vi "derive weighted array.vi"(10 "Full transition sequence from service to end":string[](array[string])=["-2 0 3 0 -3 0 4 -4 0\r\n", "0 3\r\n", "0 4 -3 0 -4 1 0 4 -3 0\r\n", "0\r\n", "-2 0 3 -3 0 -4 1 -4 0 3 -3 4 -3 0 2 0 3\r\n", "0 3 0 1\r\n", "0 1 0 3\r\n", "0 3 -2 0 4\r\n", "0\r\n", "0 -3 4 0 2 -2 0 -3 0 3 -2 3 -3 4\r\n", "0 -3 4 -3 0\r\n", "-2 0 -2 2 0\r\n", "0 3 -2\r\n", "0 4 -3 0 3 -2 0 -3 4 -3 0 3 -2 2 -2 0 4 0\r\n", "2 0 1 -4 0 3 0 -4 4 0 -4 4 0 2 0 4 0 -3 4 -3 0 -4 0 4\r\n", "0 4\r\n", "-2 0 -2 0 3 0\r\n", "0 3 0 -2 3\r\n", "0 4 0 4 -4 0 2 0 -4 4 -3 0 -2 2 -2 0 4 -3 0 2 0 3 0\r\n", "0 4 -3 0 1 -1 0 3 0 -2 2 -2 0 -3 4 -3 0 4 -4 1 0\r\n", "", "0 -3\r\n", "2 0 3 0 1 0 -2 3\r\n", "0\r\n", "1 -1 0\r\n", "0 -2 3 0\r\n", "0 1 0 4 0 4 -4 4\r\n", "0 1 -1 0 3\r\n", "0 2 -2 3 -3 4\r\n", "-2 2 0 -2 3\r\n", "0 -1\r\n", "0 4 -4 4 0 3 0 -2 0 -4 0 1 -4\r\n", "-2 0 4 0 -3 3 0 -2 2 -2 0 -4 0 4 0\r\n", "0 -1 0 -4 4 -4 1 -4 0\r\n", "1 -4 1 0 2 0 -3 0 2 0 -2 0 1 0 1 -4 4 -4 1 0 3 -2 0 -4 4 -4\r\n", "0 1 -4 4 -4 1\r\n", "0 3 0 -3 3 0 1 0 1 -4 4\r\n", "0 1 -4 0 1 -4\r\n", "0 3 -2 0 1 -4 1 0 2 0 4 0 4 0 -1 2 -1 0\r\n", "1 0 -1 0 2 0 4 -4\r\n", "-4\r\n", "-1 0 4\r\n", "0 1 -1 0 1 -4 0\r\n", "-1 0 1 -4 0 3 0 2 0 4 0 -4 4 -4 0 -1 0 -4 0 -2 0 4\r\n", "0 4 0\r\n", "0 4 -4 0 2 -1 0 2 0 4 -4 1 -4 4 0 3\r\n", "0 4 0 2 0\r\n", "1 0 -1 1 0 -4 1 -4 1 0 -4\r\n", "0 3 -2 0 -4\r\n", "2 -1 0 -4 4 -4 0 2 0 4\r\n", "1 0\r\n", "-1 0 -1 1 0 -4\r\n", "0 3 0\r\n", "0 -4 4 -4 0 -4 0 4 0 2 0 1 -4 4\r\n", "-1 0 1 -4\r\n", "-1 0 2 -1 0 2\r\n", "1 -1 0 4 -4 1\r\n", "-1 0 1 -4 4 -4 0 -4 4\r\n", "0 3 0 3 0 1 -1 0 1\r\n", "-1 0 4 0 4 -4 1 0 -4 0\r\n", "1 0 4\r\n", "0 -1 0 2 -1 0 -2 3 -2 0 -4 4 -4\r\n", "0 3 0\r\n", "2 -1 0 1 -4 4 -4 0 2 0\r\n", "0 4 -4 1 0 1 0 1 -4 0 2 0 4 0 4 -4 1\r\n", "1 -1 0 3 0 3 0 1 0 4\r\n", "0 -4 0 -2 0 -4\r\n", "0 -4 4 -4 0 -2 0 2 0\r\n", "-1 0 4 -4 0\r\n", "1 0 -1 2 0 4\r\n", "0 2 0 -2 0\r\n", "0 1 -4 0 -4 0 3 -2 0 -4 0 -4 4 -4 1\r\n", "0 4 0 4 0 4 0 4 0 -2 3 0 3 0 4 0\r\n", "-4 -1\r\n", "-2 0 1 0 -4 4\r\n", "0 4\r\n", "-2 2 0 -1 -4 1 0 3 0\r\n", "-1 0 -1 2\r\n", "0 -1 1 0 4 0 3 -2 0 -2 3 -2 0 4 0 -2 2\r\n", "2 -1 0 4\r\n", "0 4 0 2 0 -2 0\r\n", "1 -1 0 3 0 -4 4 -4 0\r\n", "2 -1 0 3 -2 0 -3 0 3 0 -3 0\r\n", "0 4 0 4 -4 1 -1 0 -3 0 1 -4 1 0 4 0 -4 0 -4 4 -4 1\r\n", "0 -4 1 0 -4 4\r\n", "0 4 0 -2 2 -2 2 -2 2\r\n", "-2 2 -1 0 4 0 2 0 4 0 2 -2 0 4\r\n", "1 0 -1 0 -1 0 1 -1\r\n", "-2 2 -2 3\r\n", "1 0 -1 0 -1 2 0 2 -2 0 -4 0\r\n", "-2 2 0 3 -2 2\r\n", "0\r\n", "1 -1 0 3\r\n", "0 4 0\r\n", "-2 0 1 -4 0 -3 0\r\n", "1 0 -1 2 -1 1 -4\r\n", "0 4\r\n", "-2 0 -1 1\r\n", "0 3 0 3 0 3 -2\r\n", "-4 0 -4 4\r\n", "0 4 0 -4 0 -4\r\n", "-2 2 0 4 -4 0 2 -2\r\n", "-2 2 -2 0 -1\r\n", "0 4 -3 0\r\n", "0 1 0 -1 1\r\n", "-4 0\r\n", "-2 0 3 0 1 0 3 -2 0 -1 0 4 0 3 0 -3 3 -3\r\n", "0 4 0 -2 0 1 0 -4 4 -3 0 1 0 4 0 -4 1 0 3 -3 0\r\n", "0 -1 2\r\n", "2 0 -3 4 0\r\n", "-4 0 -3 3 -3 0 -3 3 0 -2 3 0\r\n", "0 -1 1 -4 4 -3 0 3 0\r\n", "0 -1 2 0 3 0 1 -4 4 0 2 0\r\n", "2 -2 0 -4 0 -4 4 0 -4\r\n", "1 -1 2 -1\r\n", "2 0 -2 0 4 0 2 0 3 0 -2 0 -4\r\n", "1 -1 0 -1\r\n", "0 1 -4 1\r\n", "0 4 0 -1 1 -1 0\r\n", "0 3\r\n", "-2 0\r\n", "1 -4 0 -2 0 4 0 -4 0 4 -3 0 1 -4 0 1\r\n", "0 -3 3 -2 0 3 0 -2 2\r\n", "1 0\r\n", "2\r\n", "0 -4\r\n", "0 4 0 -4 0 -3 3 -3 0 -2 0 -2 0 4 0 -1 1 0 3 0 -4 1 -4 0 4\r\n", "2 0 -1 1\r\n", "0 2 0 4 0 4 -4 0 -1 2\r\n", "0 3 -2 0 3 -2\r\n", "1 0 -3 3 0 -4\r\n", "0 -3 3 0 -1 0\r\n", "2 -2 0 1\r\n", "-4 1 -4 1 -4 0\r\n", "0 4 0 2 0 -4 1 2 -1 0 4 0 1 0 4 -4 4 0 -4 4 0\r\n", "-2 0 3 0 -2 0\r\n"]) -> (2 "Weighted arrays":dbl[][][](array[numeric]))   [LabVIEW 2014]
panel:
  out "averaged weights":dbl[][](array[numeric])
  out "total weights":i32[][](array[numeric])
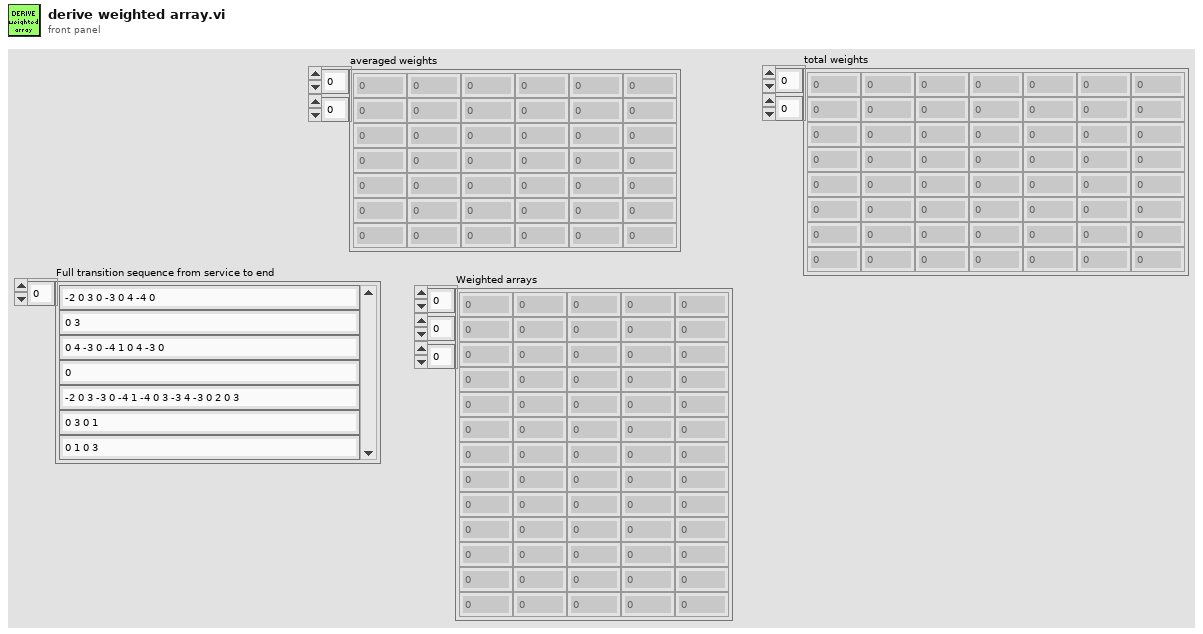
[diagram p1: front panel]
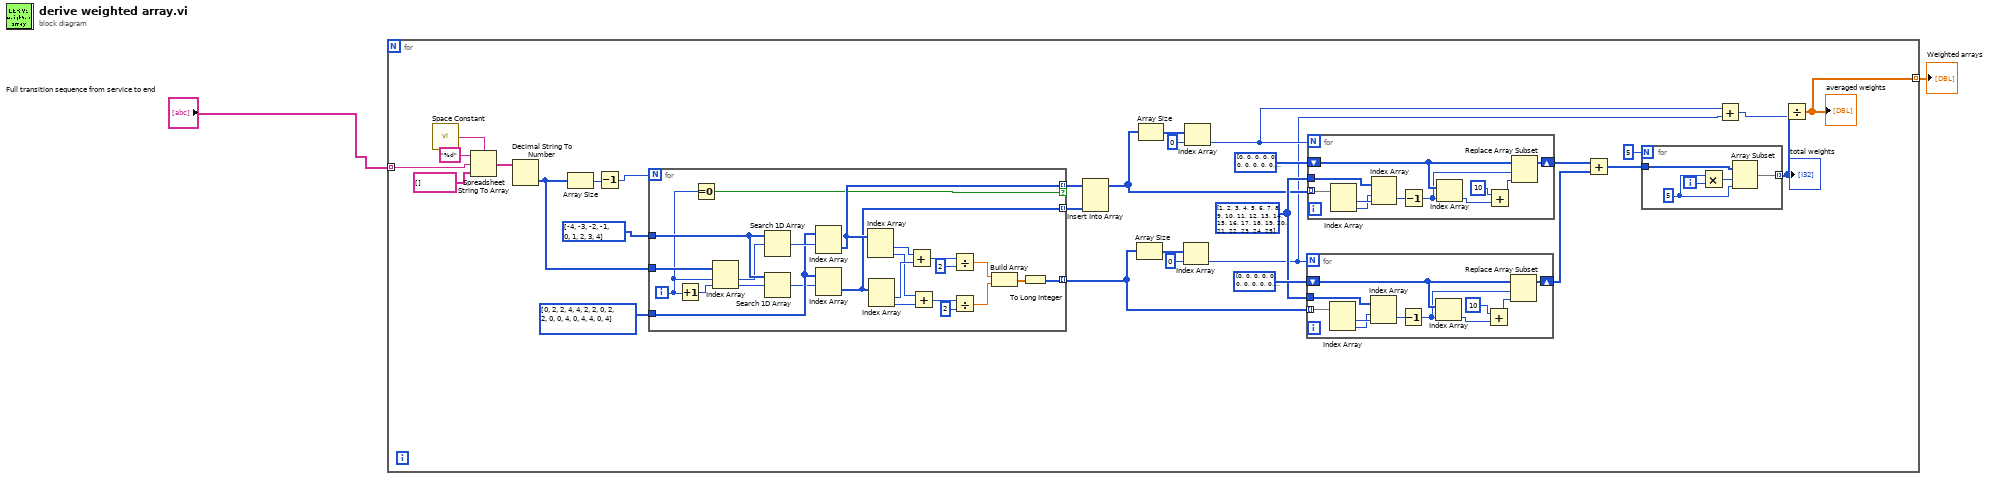
[diagram p0: block diagram]
diagram:
  n1 = for {
    tunnel: "Full transition sequence from service to end" -> [w4] mode=indexing
    tunnel: [w3] -> w1 mode=indexing
    w16 = i32[][] [[1, 2, 3, 4, 5], [6, 7, 8, 9, 10], [11, 12, 13, 14, 15], [16, 17, 18, 19, 20], [21, 22, 23, 24, 25]]
    n2 = call <vilib>:"Space Constant.vi"() -> ("String"=w32:string)
    n3 = Spreadsheet String To Array(delimiter (Tab)=w32, format string="%d", spreadsheet string=w4, array type (2D Dbl)=string[] []) -> (array=w29:string[])
    n4 = Decimal String To Number(string=w29) -> (number=w26:i32[])  [unwired: 2 in, 1 out]
    n5 = Array Size(array=w26) -> (size(s)=w28:i32)
    n6 = Decrement(x=w28) -> (x-1=w27:i32)
    n7 = for {
      N: w27 -> [_]
      tunnel: w26 -> [w82]
      tunnel: i32[] [-4, -3, -2, -1, 0, 1, 2, 3, 4] ("deleted portion") -> [w81]
      tunnel: i32[][] [[0, 2], [2, 4], [4, 2], [2, 0], [2, 2], [0, 0], [4, 0], [4, 4], [0, 4]] -> [w77]
      tunnel: [w62] -> w15 mode=indexing
      tunnel: [w63] -> w12 mode=indexing
      tunnel: [w65] -> w13 mode=indexing if=w61
      i -> [w60]
      n8 = Increment(x=w60) -> (x+1=w83:i32)
      n9 = Equal To 0?(x=w60) -> (x = 0?=w61:bool)
      n10 = Index Array(array=w82, index #1=w60, index #2=w83) -> (element #1=w80:i32, element #2=w79:i32)
      n11 = Search 1D Array(1D array=w81, element=w80) -> (index of element=w78:i32)  [unwired: 1 in]
      n12 = Search 1D Array(1D array=w81, element=w79) -> (index of element=w76:i32)  [unwired: 1 in]
      n13 = Index Array(array=w77, index (row)=w78) -> (element=w65:i32[])  [unwired: 1 in]
      n14 = Index Array(array=w77, index (row)=w76) -> (element=w63:i32[])  [unwired: 1 in]
      n15 = Index Array(array=w65) -> (element #1=w75:i32, element #2=w73:i32)  [unwired: 2 in]
      n16 = Index Array(array=w63) -> (element #1=w74:i32, element #2=w72:i32)  [unwired: 2 in]
      n17 = Add(x=w75, y=w74) -> (x+y=w71:i32)
      n18 = Add(x=w73, y=w72) -> (x+y=w68:i32)
      n19 = Divide(x=w71, y=2) -> (x/y=w67:dbl)
      n20 = Divide(x=w68, y=2) -> (x/y=w66:dbl)
      n21 = Build Array(w67, w66) -> (w64:dbl[])
      n22 = To Long Integer(number=w64) -> (32bit integer=w62:i32[])
    }
    n23 = Insert Into Array(array=w13, new element=w12) -> (w14:i32[][])  [unwired: 2 in]
    n24 = Array Size(array=w15) -> (size(s)=w18:i32[])
    n25 = Array Size(array=w14) -> (size(s)=w22:i32[])
    n26 = Index Array(array=w18, index=0) -> (element=w5:i32)
    n27 = Index Array(array=w22, index=0) -> (element=w6:i32)
    n28 = for {
      N: w5 -> [_]
      tunnel: w15 -> [w43] mode=indexing
      tunnel: w16 -> [w42]
      shift-right: [w34] -> w11
      shift-left: i32[] [0, 0, 0, 0, 0, 0, 0, 0, 0, 0, 0, 0, 0, 0, 0, 0, 0, 0, 0, 0, 0, 0, 0, 0, 0] -> [w36]
      n29 = Index Array(array=w43) -> (element #1=w41:i32, element #2=w40:i32)  [unwired: 2 in]
      n30 = Index Array(array=w42, index (row)=w40, index (col)=w41) -> (element=w39:i32)
      n31 = Decrement(x=w39) -> (x-1=w35:i32)
      n32 = Index Array(array=w36, index=w35) -> (element=w38:i32)
      n33 = Add(x=10, y=w38) -> (x+y=w37:i32)
      n34 = Replace Array Subset(array=w36, new element=w37, index=w35) -> (w34:i32[])
    }
    n35 = for {
      N: w6 -> [_]
      tunnel: w14 -> [w59] mode=indexing
      tunnel: w16 -> [w58]
      shift-right: [w50] -> w10
      shift-left: i32[] [0, 0, 0, 0, 0, 0, 0, 0, 0, 0, 0, 0, 0, 0, 0, 0, 0, 0, 0, 0, 0, 0, 0, 0, 0] -> [w52]
      n36 = Index Array(array=w59) -> (element #1=w57:i32, element #2=w56:i32)  [unwired: 2 in]
      n37 = Index Array(array=w58, index (row)=w56, index (col)=w57) -> (element=w55:i32)
      n38 = Decrement(x=w55) -> (x-1=w51:i32)
      n39 = Index Array(array=w52, index=w51) -> (element=w54:i32)
      n40 = Add(x=10, y=w54) -> (x+y=w53:i32)
      n41 = Replace Array Subset(array=w52, new element=w53, index=w51) -> (w50:i32[])
    }
    n42 = Add(x=w10, y=w11) -> (x+y=w9:i32[])
    n43 = for {
      N: 5 -> [_]
      tunnel: w9 -> [w48]
      tunnel: [w44] -> w8 mode=indexing
      i -> [w47]
      w46 = 5 ("length")
      n44 = Multiply(x=w46, y=w47) -> (x*y=w45:i32)
      n45 = Array Subset(array=w48, index=w45, length=w46) -> (w44:i32[])
    }
    "total weights" <- w8
    n46 = Add(x=w6, y=w5) -> (x+y=w7:i32)
    n47 = Divide(x=w8, y=w7) -> (x/y=w3:dbl[][])
    "averaged weights" <- w3
  }
  "Weighted arrays" <- w1
